vi "Digital module.vi"(8 "error in (no error)":errorcluster) -> (0 "error out":errorcluster)   [LabVIEW 2016]
uses:
  General/Controls/staus modes.ctl
  General/Controls/DAQ device list.ctl
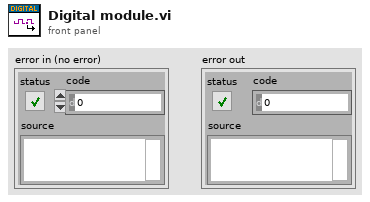
[diagram p1: front panel]
types:
  T1 = typedef "References.ctl" = cluster{"Tab Control":refnum<vi>, "Logo 1":refnum<vi>, "Logo 2":refnum<vi>, "Connect Actuator":refnum<vi>, "LIVE DATA":refnum<vi>, "Speed":refnum<vi>, "Home position":refnum<vi>, "Limit position":refnum<vi>, "Trigger":refnum<vi>, "Current position":refnum<vi>, "Connect Camera":refnum<vi>, "TEST DATA":refnum<vi>, "LIVE DATA Force":refnum<vi>, "Connect DAQ":refnum<vi>, "Initialised":refnum<vi>, "Test":refnum<vi>}
  T2 = typedef "UEs.ctl" = cluster{"Read position":refnum<user-event>, "Check home":refnum<user-event>, "Record":refnum<user-event>, "Abort controller":refnum<user-event>, "Remote test":refnum<user-event>, "Test setup":refnum<user-event>, "Conditional wait":refnum<user-event>, "Abort move":refnum<user-event>, "Wait done":refnum<user-event>, "Send trigger":refnum<user-event>, "Initalising":refnum<user-event>, "Initalisation complete":refnum<user-event>}
  T3 = typedef "staus modes.ctl" = enum16{"Status", "Testing", "Webcam", "DAQ", "Actuator", "Initialise"}
  T4 = typedef "DAQ device list.ctl" = enum16{"USB-6211", "NI myDAQ", "NI 9211"}
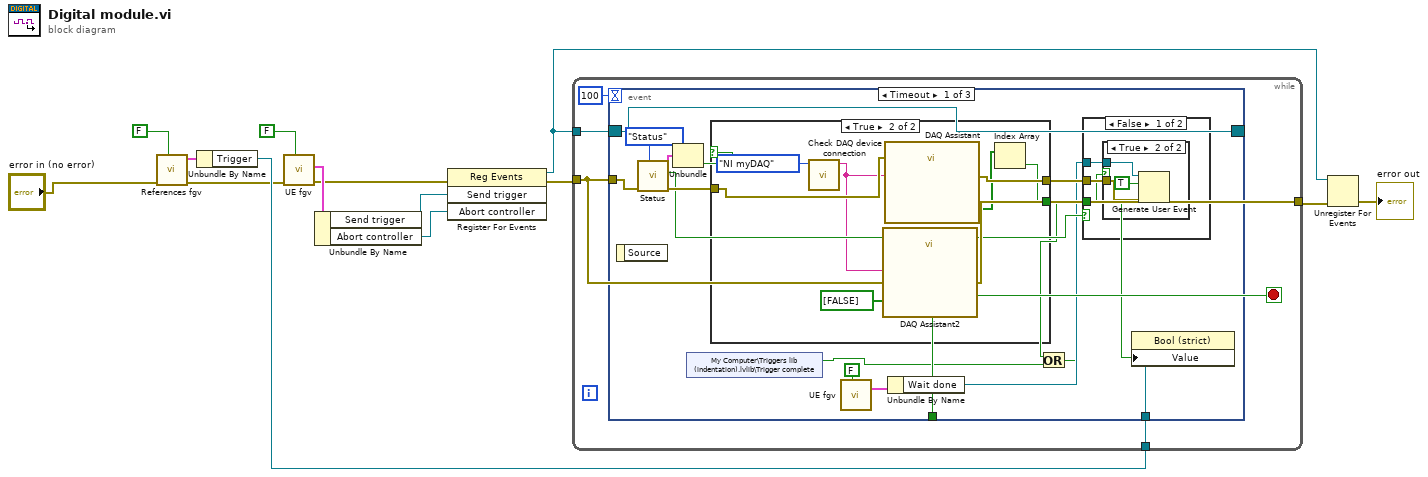
[diagram p0: block diagram]
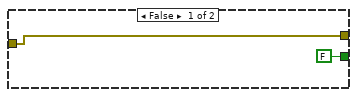
[diagram p2: hidden frame]
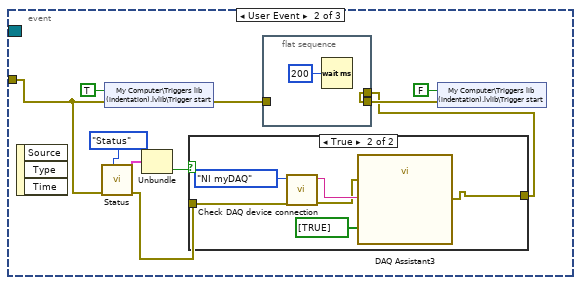
[diagram p5: hidden frame]
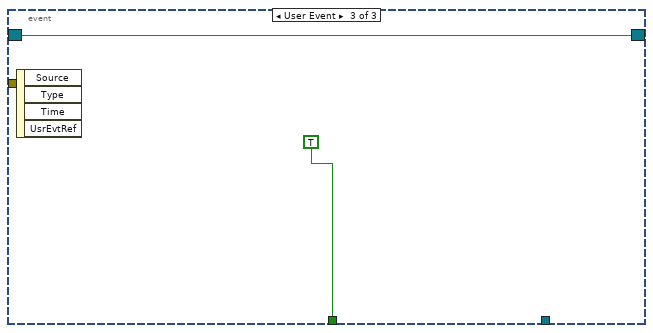
[diagram p7: hidden frame]
diagram:
  n1 = call "References fgv.vi"("Set?"=FALSE, "error in (no error)"="error in (no error)") -> ("error out"=w10:errorcluster, "Cluster"=w12:T1)  [unwired: 8 in]
  n2 = Unbundle By Name(w12) -> ("Trigger"=w11:refnum<vi>)
  n3 = call "UE fgv.vi"("Set?"=FALSE, "error in (no error)"=w10) -> ("error out"=w5:errorcluster, "UEs"=w8:T2)  [unwired: 7 in, 1 out]
  n4 = Unbundle By Name(w8) -> ("Send trigger"=w7:refnum<user-event>, "Abort controller"=w6:refnum<user-event>)
  n5 = register-events(error in=w5, w7, w6) -> (reference out=w1:refnum<event-registration>, error out=w4:errorcluster)  [unwired: 1 in]
  n6 = while {
    tunnel: w1 -> [w19]
    tunnel: [w16] -> w2
    tunnel: w4 -> [w16]
    tunnel: w11 -> [w15]
    stop <- w18 stop-if-true
    n7 = event shown="[0] Timeout" {
      selector: w19 -> [w34 _ w69]
      dyn-events: [w34 _ w69] -> _
      timeout: 100 -> [_ _ _]
      tunnel: [_ _ TRUE] -> w18
      tunnel: w16 -> [w31 w54 _]
      tunnel: w15 -> [w21 _ _]
      event Timeout {
        n8 = event-data() -> ()  [unwired: 1 in, 1 out]
        n9 = call "Status.vi"("Mode"=staus_modes."Status", "error in (no error)"=w31) -> ("error out"=w29:errorcluster, "Testing"=w27:bool, "Connections"=w33:cluster{"Data":bool, "Data":bool, "Data":bool})  [unwired: 7 in]
        n10 = Unbundle(w33) -> ("Data"=w30:bool)  [unwired: 2 out]
        n11 = shared-variable "My Computer\\Triggers lib (indentation).lvlib\\Trigger complete"() -> (w22:bool)  [unwired: 1 in, 1 out]
        n12 = case shown="True" w30 {
          tunnel: w29 -> [w36 w42]
          tunnel: [w36 w41] -> w28
          tunnel: [FALSE ("Boolean") w39] -> w23
          frame False {
          }
          frame True {
            n13 = call "Check DAQ device connection.vi"("DAQ Device"=DAQ_device_list."NI myDAQ") -> ("DAQmx Device Name"=w38:tag)  [unwired: 8 in, 2 out]
            n14 = call "DAQ Assistant2"("data"=bool[] [FALSE], "device name"=w38) -> ()  [unwired: 16 in, 2 out]
            n15 = call "DAQ Assistant"("error in"=w42, "device name"=w38) -> ("data"=w40:bool[], "error out"=w41:errorcluster)  [unwired: 15 in, 1 out]
            n16 = Index Array(array=w40) -> (element=w39:bool)  [unwired: 1 in]
          }
        }
        n17 = call "UE fgv.vi"("Set?"=FALSE) -> ("UEs"=w26:T2)  [unwired: 8 in, 2 out]
        n18 = Unbundle By Name(w26) -> ("Wait done"=w24:refnum<user-event>)
        n19 = Or(x=w23, y=w22) -> (x .or. y?=w20:bool)
        n20 = case shown="False" w27 {
          tunnel: w24 -> [w45 _]
          tunnel: w28 -> [w46 _]
          tunnel: w20 -> [w44 _]
          frame False {
            n21 = case shown="True" w44 {
              tunnel: w46 -> [_ w49]
              tunnel: w45 -> [_ w48]
              frame False {
              }
              frame True {
                n22 = Generate User Event(user event=w48, event data cluster=TRUE ("event data"), error in=w49) -> ()  [unwired: 1 in, 2 out]
              }
            }
          }
          frame True {
            # "SNAP\nIMAGE"
          }
        }
        n23 = property class="Bool (strict)"(reference=w21, "Value"=w20) -> ()  [unwired: 1 in, 2 out]
      }
      event User Event {
        n24 = event-data() -> ()  [unwired: 1 in, 3 out]
        n25 = call "Status.vi"("Mode"=staus_modes."Status", "error in (no error)"=w54) -> ("error out"=w52:errorcluster, "Connections"=w56:cluster{"Data":bool, "Data":bool, "Data":bool})  [unwired: 7 in, 1 out]
        n26 = shared-variable "My Computer\\Triggers lib (indentation).lvlib\\Trigger start"(TRUE ("Trigger start"), error in=w54) -> (error out=w50:errorcluster)
        n27 = Unbundle(w56) -> ("Data"=w53:bool)  [unwired: 2 out]
        n28 = case shown="True" w53 {
          tunnel: w52 -> [w60 w65]
          tunnel: [w60 w61] -> w51
          frame False {
          }
          frame True {
            n29 = call "Check DAQ device connection.vi"("error in (no error)"=w65, "DAQ Device"=DAQ_device_list."NI myDAQ") -> ("error out"=w62:errorcluster, "DAQmx Device Name"=w63:tag)  [unwired: 7 in, 1 out]
            n30 = call "DAQ Assistant3"("data"=bool[] [TRUE], "error in"=w62, "device name"=w63) -> ("error out"=w61:errorcluster)  [unwired: 15 in, 1 out]
          }
        }
        n31 = flat-sequence {
          tunnel: [w67] -> w59
          tunnel: w51 -> [w67]
          tunnel: w50 -> [_]
          frame #0 {
            n32 = Wait (ms)(milliseconds to wait=u32 200) -> ()  [unwired: 1 out]
          }
        }
        n33 = shared-variable "My Computer\\Triggers lib (indentation).lvlib\\Trigger start"(FALSE ("Trigger start"), error in=w59) -> ()  [unwired: 1 out]
      }
      event User Event {
        n34 = event-data() -> ()  [unwired: 1 in, 4 out]
      }
    }
  }
  n35 = Unregister For Events(event registration refnum=w1, error in=w2) -> (error out=→"error out":errorcluster)
